vi "Write to Cluster.vi"(6 "Tag Cluster.Time Stamp":timestamp, 7 "AMQP":bool, 8 "Skylink Index":i32, 9 "String":string, 10 "HTTP  in":T1[](array[typedef]), 11 "AMQP  in":T1[](array[typedef])) -> (2 "HTTP  out":T1[](array[typedef]), 3 "AMQP  out":T1[](array[typedef]))   [LabVIEW 2015, in "SystemLink File runtime.lvclass"]
uses:
  SystemLink File runtime.lvclass
  <vilib>/Skyline/Tag/Wrapper/Wrapper_class/Tag Value Cluster Wrapper.ctl
  <vilib>/Skyline/Configuration/Configuration_class/NI Skyline Configuration.lvclass
  <vilib>/Skyline/Tag/Shared/typedefs/Tag Value Cluster.ctl
  <vilib>/Skyline/Tag/Shared/typedefs/DataType.ctl
  <vilib>/Skyline/Tag/Shared/NI Skyline Tag.lvlib
  <vilib>/Skyline/Tag/Wrapper/Wrapper_class/NI Skyline Tag.lvclass
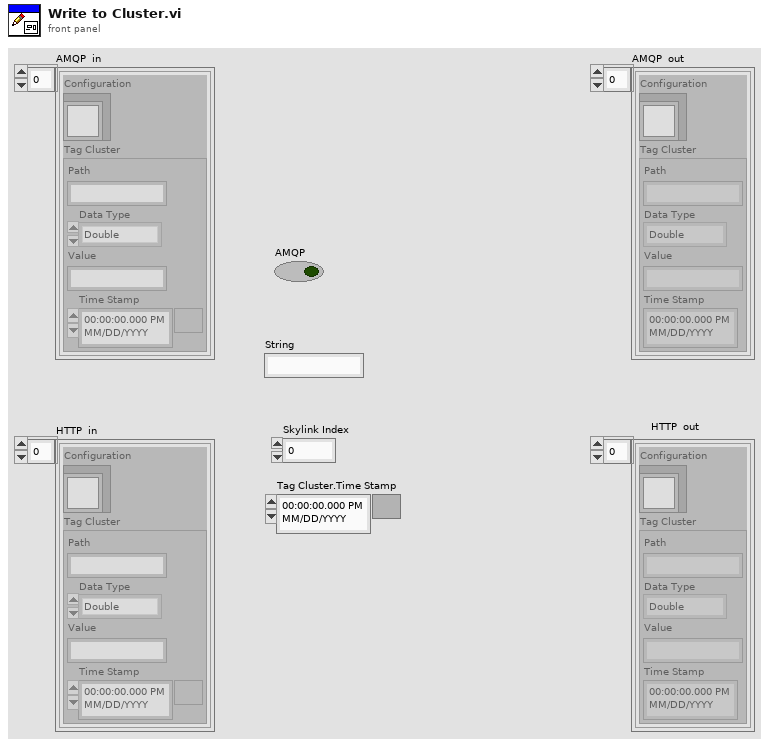
[diagram p1: front panel]
types:
  T1 = typedef "NI Skyline Tag.lvclass/Tag Value Cluster Wrapper.ctl" = cluster{"Configuration":refnum<class "NI Skyline Configuration.lvclass">, "Tag Cluster":T2}
  T2 = typedef "NI Skyline Tag.lvlib/Tag Value Cluster.ctl" = cluster{"Path":string, "Data Type":T3, "Value":string, "Time Stamp":timestamp}
  T3 = typedef "NI Skyline Tag.lvlib/DataType.ctl" = enum32{"Double", "I32", "String", "Boolean", "U64", "Timestamp"}
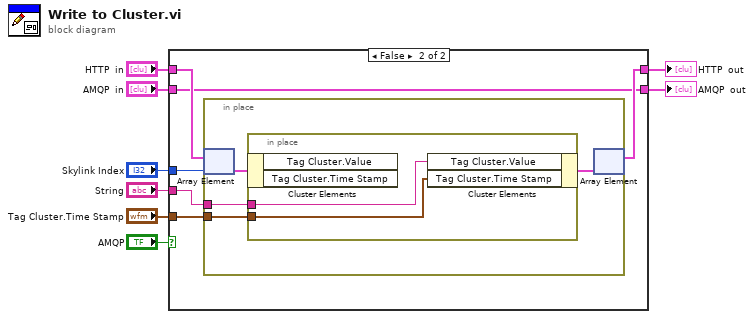
[diagram p0: block diagram]
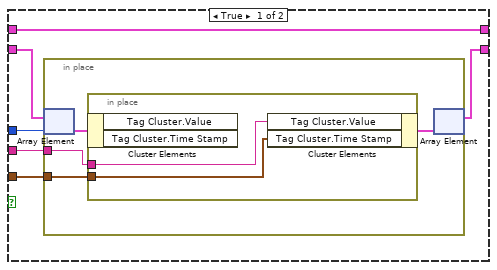
[diagram p2: hidden frame]
diagram:
  n1 = case shown="False" "AMQP" {
    tunnel: "AMQP  in" -> [w14 w21]
    tunnel: "Skylink Index" -> [w13 w26]
    tunnel: [w12 w21] -> w5
    tunnel: [w11 w22] -> w6
    tunnel: "HTTP  in" -> [w11 w23]
    tunnel: "String" -> [w10 w25]
    tunnel: "Tag Cluster.Time Stamp" -> [w9 w24]
    frame True {
      n2 = in-place {
        in-place-border: w10 -> [w15]
        in-place-border: w9 -> [w16]
        n3 = in-place-array #1(w14, w13) -> (w18:T1)
        n4 = in-place {
          in-place-border: w16 -> [w20]
          in-place-border: w15 -> [w19]
          n5 = in-place-cluster #2(w18) -> ()  [unwired: 2 out]
          n6 = in-place-cluster #2("Tag Cluster.Value"=w19, "Tag Cluster.Time Stamp"=w20) -> (w17:T1)
        }
        n7 = in-place-array #1(w17) -> (w12:T1[])  [unwired: 1 out]
      }
    }
    frame False {
      n8 = in-place {
        in-place-border: w25 -> [w27]
        in-place-border: w24 -> [w28]
        n9 = in-place-array #3(w23, w26) -> (w30:T1)
        n10 = in-place {
          in-place-border: w28 -> [w32]
          in-place-border: w27 -> [w31]
          n11 = in-place-cluster #4(w30) -> ()  [unwired: 2 out]
          n12 = in-place-cluster #4("Tag Cluster.Value"=w31, "Tag Cluster.Time Stamp"=w32) -> (w29:T1)
        }
        n13 = in-place-array #3(w29) -> (w22:T1[])  [unwired: 1 out]
      }
    }
  }
  "HTTP  out" <- w6
  "AMQP  out" <- w5
